vi "CaptureImage.vi"(0 "Camera":T1="cam1", 1 "Rotate (degrees)":sgl, 2 "ImageName":string="name1", 3 "Draw50MicroCircleAtCenter":bool, 5 "error in (no error)":errorcluster) -> (6 "Image":T2(plugin-control), 8 "error out":errorcluster)   [LabVIEW 2019]
uses:
  <vilib>/userDefined/High Color/IMAQdx.ctl
  <vilib>/vision/driver/NI_Vision_Acquisition_Software.lvlib
  <vilib>/vision/NI_Vision_Development_Module.lvlib
panel:
  in  "CircleRadiusPixels":dbl=73.28
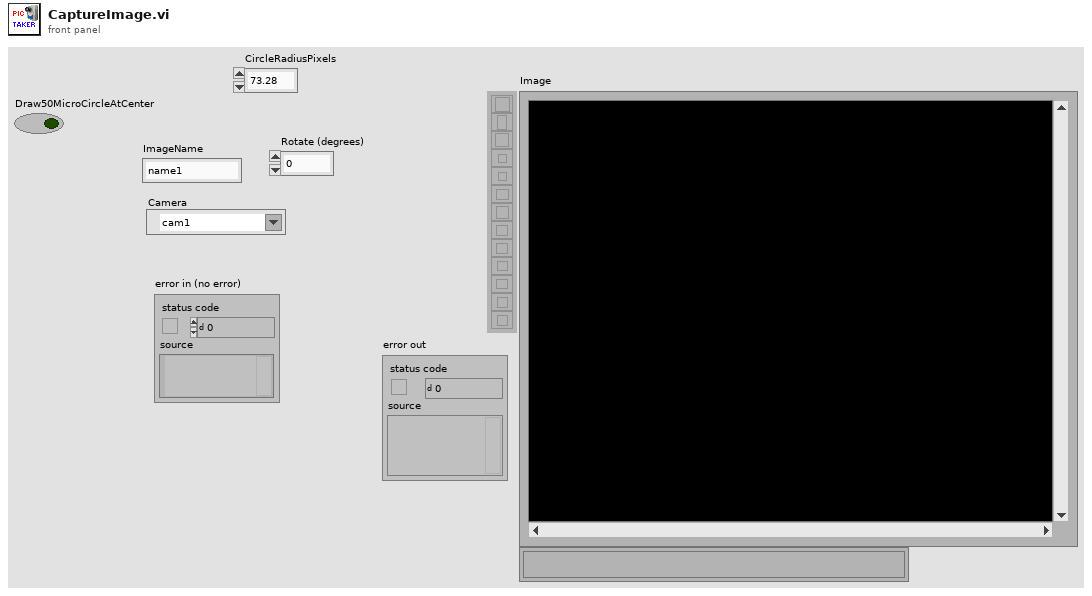
[diagram p1: front panel]
types:
  T1 = typedef "IMAQdx.ctl" = refnum<k21>
  T2 = typedef "IMAQ Image.ctl" = refnum<image>
  T3 = typedef "Image Type" = u32
  T4 = typedef "IMAQ Circle" = cluster{"Center X":i32, "Center Y":i32, "Inner Radius":i32, "Outer Radius":i32, "Start Angle":dbl, "End Angle":dbl}
  T5 = typedef "ROI Descriptor" = cluster{"Global Rectangle":i32[], "Contours":cluster{"ID":enum32{"External", "Internal"}, "Type":u32, "Coordinates":i32[]}[]}
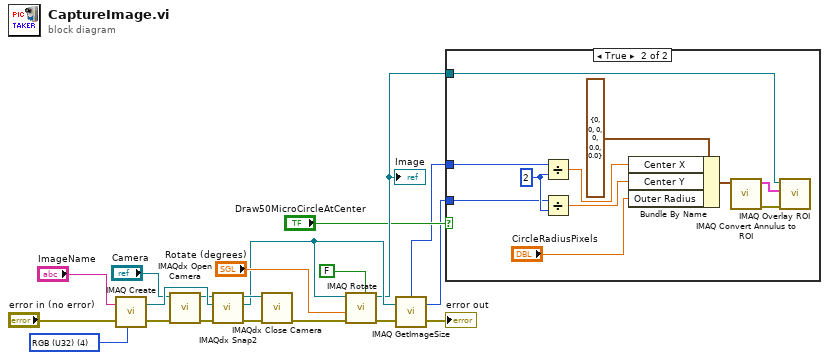
[diagram p0: block diagram]
diagram:
  w18 = T3 4 items=["Grayscale (U8)", "Grayscale (I16)", "Grayscale (SGL)", "Complex (CSG)", "RGB (U32)", "HSL (U32)", "RGB (U64)", "Grayscale (U16)"] ("Image Type")
  n1 = call "IMAQ Create"("Image Name"="ImageName", "Image Type"=w18, "error in (no error)"="error in (no error)") -> ("New Image"=w20:T2, "error out"=w19:errorcluster)  [unwired: 2 in]
  n2 = call <vilib>:"IMAQdx Open Camera.vi"("error in"=w19, "Session In"="Camera") -> ("error out"=w13:errorcluster, "Session Out"=w12:T1)  [unwired: 8 in]
  n3 = call <vilib>:"IMAQdx Snap2.vi"("error in"=w13, "Image In"=w20, "Session In"=w12) -> ("error out"=w2:errorcluster, "Image Out"=w9:T2, "Session Out"=w14:T1)  [unwired: 6 in]
  n4 = call <vilib>:"IMAQdx Close Camera.vi"("error in"=w2, "Session In"=w14) -> ("error out"=w8:errorcluster)  [unwired: 9 in]
  n5 = call "IMAQ Rotate"("Maintain Size"=FALSE, "error in (no error)"=w8, "Angle (degrees)"="Rotate (degrees)", "Image Src"=w9) -> ("error out"=w5:errorcluster, "Image Dst Out"=w7:T2)  [unwired: 6 in]
  "Image" <- w7
  n6 = call "IMAQ GetImageSize"("Image"=w9, "error in (no error)"=w5) -> ("Y Resolution"=w4:i32, "X Resolution"=w3:i32, "error out"=→"error out":errorcluster)  [unwired: 2 in]
  n7 = case shown="True" "Draw50MicroCircleAtCenter" {
    tunnel: w7 -> [_ w26]
    tunnel: w4 -> [_ w24]
    tunnel: w3 -> [_ w23]
    frame False {
    }
    frame True {
      w25 = 2 ("y")
      n8 = Divide(x=w23, y=w25) -> (x/y=w21:dbl)
      n9 = Divide(x=w24, y=w25) -> (x/y=w22:dbl)
      n10 = Bundle By Name(cluster=T4 {"Center X"=0, "Center Y"=0, "Inner Radius"=0, "Outer Radius"=0, "Start Angle"=0.0, "End Angle"=0.0} ("Annulus"), "Center X"=w21, "Center Y"=w22, "Outer Radius"="CircleRadiusPixels") -> (w31:T4)
      n11 = call "IMAQ Convert Annulus to ROI"("Annulus"=w31) -> ("error out"=w30:errorcluster, "ROI Descriptor"=w29:T5)  [unwired: 8 in]
      n12 = call "IMAQ Overlay ROI"("error in (no error)"=w30, "ROI Descriptor"=w29, "Image"=w26) -> ()  [unwired: 7 in, 2 out]
    }
  }
